vi "Set Parameter Definition.vi"(8 "error in":errorcluster, 10 "parameter definition":T1, 11 "parameter in":T2 format="%.0x") -> (0 "error out":errorcluster, 3 "parameter out":T2 format="%.0x")   [LabVIEW 2020, in "AIM MIL-STD-1553 Scripting.lvlib"]
uses:
  AIM MIL-STD-1553 Scripting.lvlib
  Constants.vi
  <vilib>/NI VeriStand/Custom Device API/Custom Device API.lvlib
  <vilib>/NI VeriStand/Custom Device API/Set Item Property (I32).vi
  <vilib>/NI VeriStand/Custom Device API/Set Item Property (U16).vi
  <vilib>/NI VeriStand/Custom Device API/Set Item Property (Boolean).vi
  <vilib>/NI VeriStand/Custom Device API/Set Item Property (Double).vi
  <vilib>/NI VeriStand/Custom Device API/Custom Device Item Ref.ctl
  Shared/Parameter Definition.ctl
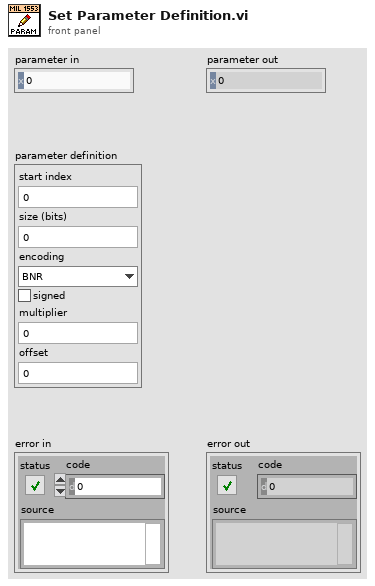
[diagram p1: front panel]
types:
  T1 = typedef "Parameter Definition.ctl" = cluster{"start index":i32, "size (bits)":i32, "encoding":enum16{"BNR", "BCD", "Discrete"}, "signed":bool, "multiplier":dbl, "offset":dbl}
  T2 = typedef "Custom Device API.lvlib/Custom Device Item Ref.ctl" = u64
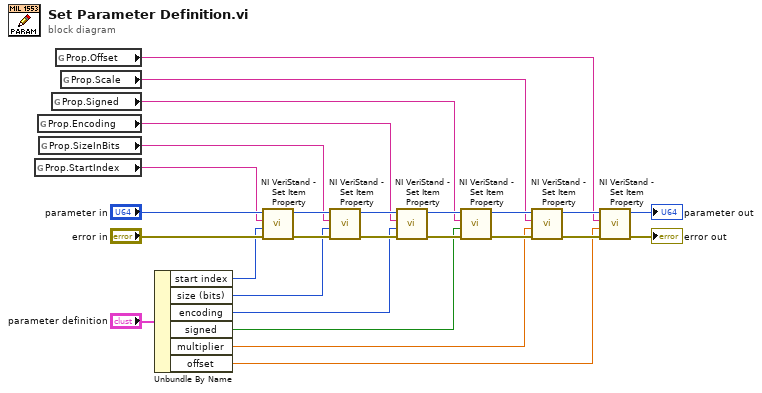
[diagram p0: block diagram]
diagram:
  n1 = global read "Constants.vi" "Prop.StartIndex"() -> (w8:string)
  n2 = global read "Constants.vi" "Prop.Encoding"() -> (w10:string)
  n3 = global read "Constants.vi" "Prop.SizeInBits"() -> (w9:string)
  n4 = global read "Constants.vi" "Prop.Signed"() -> (w11:string)
  n5 = global read "Constants.vi" "Prop.Offset"() -> (w13:string)
  n6 = global read "Constants.vi" "Prop.Scale"() -> (w12:string)
  n7 = Unbundle By Name("parameter definition") -> ("start index"=w6:i32, "size (bits)"=w5:i32, "encoding"=w4:enum16{"BNR", "BCD", "Discrete"}, "signed"=w3:bool, "multiplier"=w2:dbl, "offset"=w1:dbl)
  n8 = call-poly <vilib>:"NI VeriStand - Set Item Property.vi"("error in (no error)"="error in", "Value"=w6, "Property Name"=w8, "Item Ref in"="parameter in") -> ("error out"=w26:errorcluster, "Item Ref out"=w27:T2)  [unwired: 5 in, 1 out]
  n9 = call-poly <vilib>:"NI VeriStand - Set Item Property.vi"("error in (no error)"=w26, "Value"=w5, "Property Name"=w9, "Item Ref in"=w27) -> ("error out"=w24:errorcluster, "Item Ref out"=w25:T2)  [unwired: 5 in, 1 out]
  n10 = call-poly <vilib>:"NI VeriStand - Set Item Property.vi"("error in (no error)"=w24, "Value"=w4, "Property Name"=w10, "Item Ref in"=w25) -> ("error out"=w22:errorcluster, "Item Ref out"=w23:T2)  [unwired: 5 in, 1 out]
  n11 = call-poly <vilib>:"NI VeriStand - Set Item Property.vi"("error in (no error)"=w22, "Value"=w3, "Property Name"=w11, "Item Ref in"=w23) -> ("error out"=w20:errorcluster, "Item Ref out"=w21:T2)  [unwired: 5 in, 1 out]
  n12 = call-poly <vilib>:"NI VeriStand - Set Item Property.vi"("error in (no error)"=w20, "Value"=w2, "Property Name"=w12, "Item Ref in"=w21) -> ("error out"=w18:errorcluster, "Item Ref out"=w19:T2)  [unwired: 5 in, 1 out]
  n13 = call-poly <vilib>:"NI VeriStand - Set Item Property.vi"("error in (no error)"=w18, "Value"=w1, "Property Name"=w13, "Item Ref in"=w19) -> ("error out"=→"error out":errorcluster, "Item Ref out"=→"parameter out":T2)  [unwired: 5 in, 1 out]
